vi "Finding Numbers Within a User Defined Range of an Array 2012 NIVerified.vi"() -> ()   [LabVIEW 2017]
panel:
  out "Sub-Array Size":i32
  out "Sorted Sub Array between Min and Max Values":dbl[](array[numeric])
  in  "Min Value":dbl
  in  "Max Value":dbl=1000.0
  out "100 Random Numbers (0-1000)":dbl[](array[numeric])
  # "Overview:Filter array elements between a specified minimum and maximum value.\nRequirements:\n•\tLabVIEW 2012 (or compatible)\nInstructions:\n•\tConfigure the desired \"Min Value\" and \"Max Value\"\n•\tRun the program"
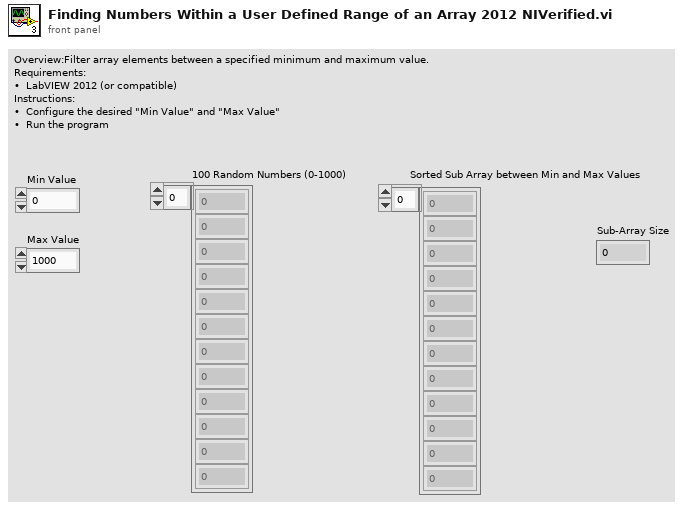
[diagram p1: front panel]
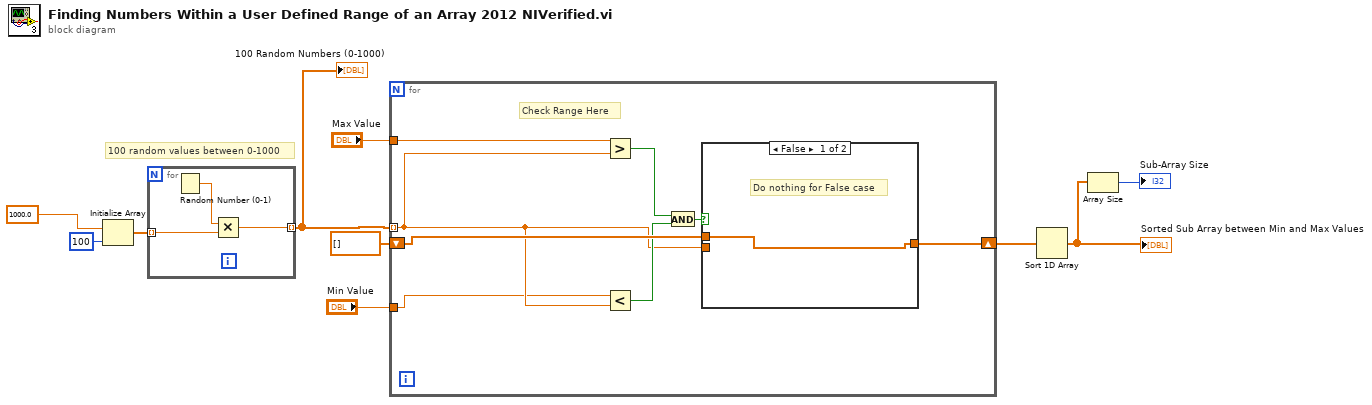
[diagram p0: block diagram]
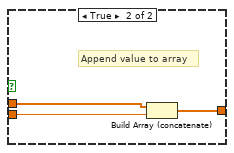
[diagram p2: hidden frame]
diagram:
  # "100 random values between 0-1000"
  n1 = Initialize Array(1000.0 ("element"), 100 ("dimension size")) -> (w7:dbl[])
  n2 = for {
    tunnel: w7 -> [w13] mode=indexing
    tunnel: [w12] -> w6 mode=indexing
    n3 = Random Number (0-1)() -> (number: 0 to 1=w11:dbl)
    n4 = Multiply(x=w11, y=w13) -> (x*y=w12:dbl)
  }
  "100 Random Numbers (0-1000)" <- w6
  n5 = for {
    tunnel: w6 -> [w16] mode=indexing
    shift-right: [w21] -> w10
    shift-left: dbl[] [] -> [w20]
    tunnel: "Max Value" -> [w15]
    tunnel: "Min Value" -> [w14]
    # "Check Range Here"
    n6 = Greater?(x=w15, y=w16) -> (0:w18:bool)
    n7 = Less?(x=w14, y=w16) -> (x < y?=w17:bool)
    n8 = And(x=w18, y=w17) -> (x .and. y?=w19:bool)
    n9 = case shown="False" w19 {
      tunnel: [w22 w25] -> w21
      tunnel: w16 -> [_ w24]
      tunnel: w20 -> [w22 w23]
      frame False {
        # "Do nothing for False case"
      }
      frame True {
        # "Append value to array"
        n10 = Build Array (concatenate)(w23, w24) -> (w25:dbl[])
      }
    }
  }
  n11 = Sort 1D Array(array=w10) -> (sorted array=w4:dbl[])
  "Sorted Sub Array between Min and Max Values" <- w4
  n12 = Array Size(array=w4) -> (size(s)=→"Sub-Array Size":i32)
